vi "标样核查.vi"(11 "标样核查配置":T1={"数据保存间隔"=1.0, "水温标样值"=0.0, "pH标样值"=0.0, "溶解氧标样值"=0.0, "电导率标样值"=0.0, "浊度标样值"=0.0}) -> ()   [LabVIEW 2016, in "斯坦道多参数.lvlib"]
panel:
  out "运行状态":u16(ring) items=["空闲", "水样测试", "标样核查"]
  out "seconds since 1Jan1904":timestamp
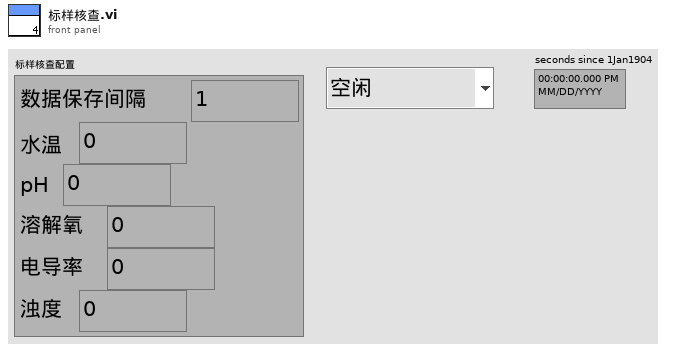
[diagram p1: front panel]
types:
  T1 = cluster{"数据保存间隔":dbl, "水温标样值":dbl, "pH标样值":dbl, "溶解氧标样值":dbl, "电导率标样值":dbl, "浊度标样值":dbl}
  T2 = cluster{"因子编码":string, "单位":string, "标样参考值":sgl, "水样数据时间":timestamp, "水样实测值":sgl, "水样数据标识":string, "探头温度":sgl}
  T3 = typedef "LVDateTimeRec.ctl" = cluster{"秒数的小数部分":dbl, "秒":i32, "分":i32, "时":i32, "日":i32, "月":i32, "年":i32, "天数（周）":i32, "天数（年）":i32, "DST":i32}
  T4 = cluster{"温度测量值":sgl, "DO%":sgl, "DOmg/L":sgl, "温度偏移修正值":sgl}
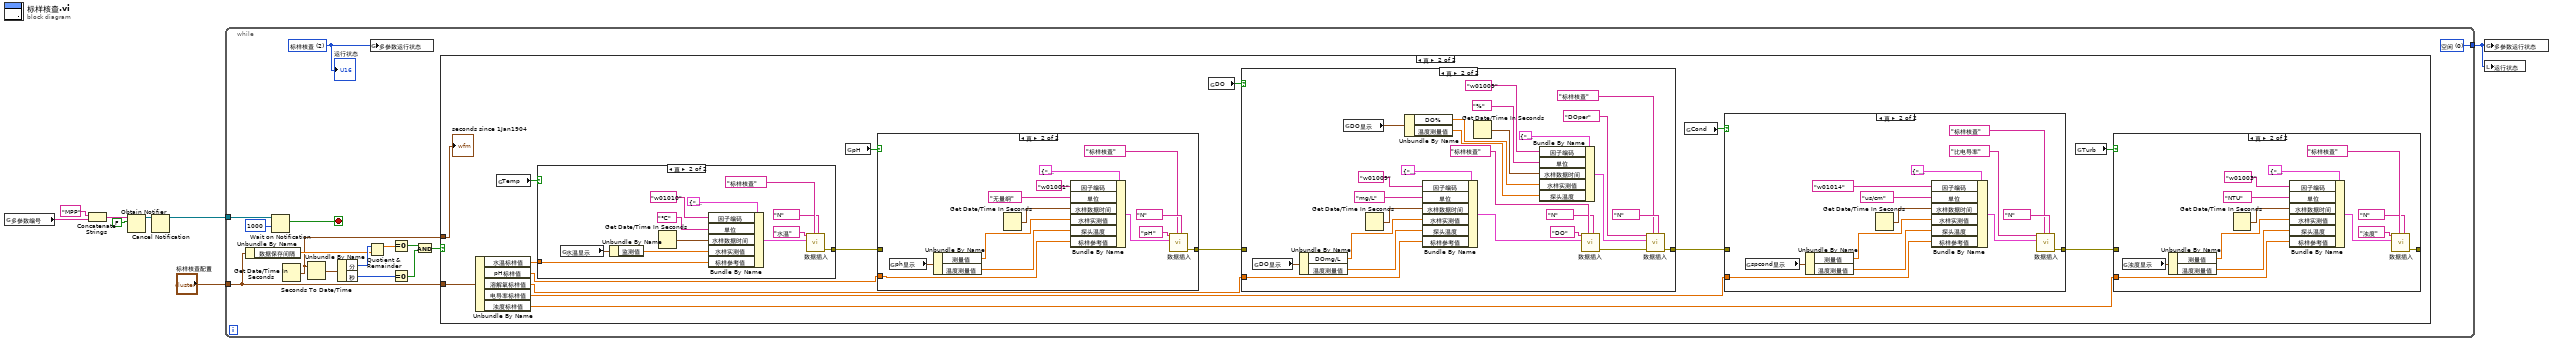
[diagram p0: block diagram]
diagram:
  n1 = global read "多参数全局变量.vi" "多参数编号"() -> (w1:string)
  n2 = Concatenate Strings("MPP" ("名称（未命名）"), w1) -> (w2:string)
  n3 = Obtain Notifier(name (unnamed)=w2, notification data type=FALSE) -> (notifier out=w5:refnum<notifier>)  [unwired: 2 in, 2 out]
  n4 = Cancel Notification(0:w5) -> (8:w4:refnum<notifier>)  [unwired: 1 in, 2 out]
  n5 = while {
    tunnel: "标样核查配置" -> [w19]
    tunnel: [w13] -> w3
    tunnel: w4 -> [w12]
    stop <- w10 stop-if-true
    w13 = u16 0 items=["空闲", "水样测试", "标样核查"] ("多参数运行状态")
    w9 = u16 2 items=["空闲", "水样测试", "标样核查"] ("多参数运行状态")
    n6 = Unbundle By Name(w19) -> ("数据保存间隔"=w17:dbl)
    n7 = Wait on Notification(notifier=w12, timeout in ms (-1)=1000 ("超时毫秒(-1)")) -> (notification=w10:bool)  [unwired: 2 in, 3 out]
    n8 = Get Date/Time In Seconds() -> (seconds since 1Jan1904=w14:timestamp)
    n9 = Seconds To Date/Time(time stamp (now)=w14) -> (date time rec=w23:T3)  [unwired: 1 in]
    n10 = Unbundle By Name(w23) -> ("分"=w18:i32, "秒"=w22:i32)
    n11 = Quotient & Remainder(x=w18, y=w17) -> (x-y*floor(x/y)=w16:dbl)  [unwired: 1 out]
    n12 = global write "多参数全局变量.vi" "多参数运行状态"(w9) -> ()
    n13 = Equal To 0?(x=w16) -> (x = 0?=w15:bool)
    n14 = Equal To 0?(x=w22) -> (x = 0?=w21:bool)
    n15 = And(x=w15, y=w21) -> (x .and. y?=w20:bool)
    n16 = case shown="真" w20 {
      tunnel: w19 -> [_ w29]
      tunnel: w14 -> [_ w39]
      frame False {
      }
      frame True {
        n17 = Unbundle By Name(w29) -> ("水温标样值"=w28:dbl, "pH标样值"=w27:dbl, "溶解氧标样值"=w26:dbl, "电导率标样值"=w25:dbl, "浊度标样值"=w24:dbl)
        n18 = global read "断电保存变量.vi" "Temp"() -> (w34:bool)
        n19 = case shown="真" w34 {
          tunnel: [_ w107] -> w38
          tunnel: w28 -> [_ w106]
          frame False {
          }
          frame True {
            n20 = global read "多参数全局变量.vi" "水温显示"() -> (w105:cluster{"CH":u16, "监测值":dbl, "温度偏移修正值":sgl})
            n21 = Unbundle By Name(w105) -> ("监测值"=w104:dbl)
            n22 = Get Date/Time In Seconds() -> (seconds since 1Jan1904=w114:timestamp)
            n23 = Bundle By Name(cluster=T2 {"因子编码"="w01003", "单位"="无量纲", "标样参考值"=0.0, "水样数据时间"=timestamp(0 s since 1904-01-01), "水样实测值"=0.0, "水样数据标识"="N", "探头温度"=0.0} ("data in"), "因子编码"="w01010", "单位"="℃", "水样数据时间"=w114, "水样实测值"=w104, "标样参考值"=w106) -> (w113:T2)
            n24 = call "数据插入.vi"("数据标记表"="N", "测量模式"="标样核查", "data in"=w113, "table输入"="水温") -> ("error out"=w107:errorcluster)  [unwired: 7 in]
          }
        }
        n25 = global read "断电保存变量.vi" "pH"() -> (w33:bool)
        n26 = case shown="真" w33 {
          tunnel: w38 -> [_ _]
          tunnel: [_ w95] -> w37
          tunnel: w27 -> [_ w94]
          frame False {
          }
          frame True {
            n27 = global read "多参数全局变量.vi" "ph显示"() -> (w93:cluster{"温度测量值":sgl, "测量值":sgl, "温度偏移修正值":sgl})
            n28 = Unbundle By Name(w93) -> ("测量值"=w92:sgl, "温度测量值"=w91:sgl)
            n29 = Get Date/Time In Seconds() -> (seconds since 1Jan1904=w100:timestamp)
            n30 = Bundle By Name(cluster=T2 {"因子编码"="w01003", "单位"="无量纲", "标样参考值"=0.0, "水样数据时间"=timestamp(0 s since 1904-01-01), "水样实测值"=0.0, "水样数据标识"="N", "探头温度"=0.0} ("data in"), "因子编码"="w01001", "单位"="无量纲", "水样数据时间"=w100, "水样实测值"=w92, "探头温度"=w91, "标样参考值"=w94) -> (w101:T2)
            n31 = call "数据插入.vi"("数据标记表"="N", "测量模式"="标样核查", "data in"=w101, "table输入"="pH") -> ("error out"=w95:errorcluster)  [unwired: 7 in]
          }
        }
        n32 = global read "断电保存变量.vi" "DO"() -> (w32:bool)
        n33 = case shown="真" w32 {
          tunnel: w37 -> [_ _]
          tunnel: [_ w78] -> w36
          tunnel: w26 -> [_ w80]
          frame False {
          }
          frame True {
            n34 = global read "多参数全局变量.vi" "DO显示"() -> (w66:T4)
            n35 = Unbundle By Name(w66) -> ("DOmg/L"=w88:sgl, "温度测量值"=w90:sgl)
            n36 = global read "多参数全局变量.vi" "DO显示"() -> (w67:T4)
            n37 = Get Date/Time In Seconds() -> (seconds since 1Jan1904=w87:timestamp)
            n38 = Unbundle By Name(w67) -> ("DO%"=w71:sgl, "温度测量值"=w69:sgl)
            n39 = Bundle By Name(cluster=T2 {"因子编码"="w01003", "单位"="无量纲", "标样参考值"=0.0, "水样数据时间"=timestamp(0 s since 1904-01-01), "水样实测值"=0.0, "水样数据标识"="N", "探头温度"=0.0} ("data in"), "因子编码"="w01009", "单位"="mg/L", "水样数据时间"=w87, "水样实测值"=w88, "探头温度"=w90, "标样参考值"=w80) -> (w86:T2)
            n40 = Get Date/Time In Seconds() -> (seconds since 1Jan1904=w72:timestamp)
            n41 = Bundle By Name(cluster=T2 {"因子编码"="w01003", "单位"="无量纲", "标样参考值"=0.0, "水样数据时间"=timestamp(0 s since 1904-01-01), "水样实测值"=0.0, "水样数据标识"="N", "探头温度"=0.0} ("data in"), "因子编码"="w01009", "单位"="%", "水样数据时间"=w72, "水样实测值"=w71, "探头温度"=w69) -> (w68:T2)
            n42 = call "数据插入.vi"("数据标记表"="N", "测量模式"="标样核查", "data in"=w86, "table输入"="DO") -> ("error out"=w79:errorcluster)  [unwired: 7 in]
            n43 = call "数据插入.vi"("数据标记表"="N", "测量模式"="标样核查", "error in (no error)"=w79, "data in"=w68, "table输入"="DOper") -> ("error out"=w78:errorcluster)  [unwired: 6 in]
          }
        }
        n44 = global read "断电保存变量.vi" "Cond"() -> (w31:bool)
        n45 = case shown="真" w31 {
          tunnel: w36 -> [_ _]
          tunnel: [_ w57] -> w35
          tunnel: w25 -> [_ w56]
          frame False {
          }
          frame True {
            n46 = global read "多参数全局变量.vi" "spcond显示"() -> (w55:cluster{"温度测量值":sgl, "测量值":sgl, "温度偏移修正值":sgl})
            n47 = Unbundle By Name(w55) -> ("测量值"=w54:sgl, "温度测量值"=w53:sgl)
            n48 = Get Date/Time In Seconds() -> (seconds since 1Jan1904=w62:timestamp)
            n49 = Bundle By Name(cluster=T2 {"因子编码"="w01003", "单位"="无量纲", "标样参考值"=0.0, "水样数据时间"=timestamp(0 s since 1904-01-01), "水样实测值"=0.0, "水样数据标识"="N", "探头温度"=0.0} ("data in"), "因子编码"="w01014", "单位"="us/cm", "水样数据时间"=w62, "水样实测值"=w54, "探头温度"=w53, "标样参考值"=w56) -> (w63:T2)
            n50 = call "数据插入.vi"("数据标记表"="N", "测量模式"="标样核查", "data in"=w63, "table输入"="比电导率") -> ("error out"=w57:errorcluster)  [unwired: 7 in]
          }
        }
        n51 = global read "断电保存变量.vi" "Turb"() -> (w30:bool)
        n52 = case shown="真" w30 {
          tunnel: w35 -> [_ _]
          tunnel: [_ w44] -> _
          tunnel: w24 -> [_ w43]
          frame False {
          }
          frame True {
            n53 = global read "多参数全局变量.vi" "浊度显示"() -> (w42:cluster{"温度测量值":sgl, "测量值":sgl, "温度偏移修正值":sgl})
            n54 = Unbundle By Name(w42) -> ("测量值"=w41:sgl, "温度测量值"=w40:sgl)
            n55 = Get Date/Time In Seconds() -> (seconds since 1Jan1904=w51:timestamp)
            n56 = Bundle By Name(cluster=T2 {"因子编码"="w01003", "单位"="无量纲", "标样参考值"=0.0, "水样数据时间"=timestamp(0 s since 1904-01-01), "水样实测值"=0.0, "水样数据标识"="N", "探头温度"=0.0} ("data in"), "因子编码"="w01003", "单位"="NTU", "水样数据时间"=w51, "水样实测值"=w41, "探头温度"=w40, "标样参考值"=w43) -> (w50:T2)
            n57 = call "数据插入.vi"("数据标记表"="N", "测量模式"="标样核查", "data in"=w50, "table输入"="浊度") -> ("error out"=w44:errorcluster)  [unwired: 7 in]
          }
        }
        "seconds since 1Jan1904" <- w39
      }
    }
    "运行状态" <- w9
  }
  n58 = global write "多参数全局变量.vi" "多参数运行状态"(w3) -> ()
  n59 = local write "运行状态"(w3) -> ()
